vi "Data Tag Type to SysLink Type.vi"(11 "Data Tag Type":T2) -> (3 "data type":T1=enum."U64" caption="Systeme Link Data Type")   [LabVIEW 2015, in "SystemLink File configuration.lvclass"]
doc: "Converts Data Tag Type.ctl to the correct System Link data type. This is used to convert the user selected data type to a data type that system link can use."
uses:
  SystemLink File configuration.lvclass
  Data Tag Type.ctl
  <vilib>/Skyline/Tag/Shared/typedefs/DataType.ctl
  <vilib>/Skyline/Tag/Shared/NI Skyline Tag.lvlib
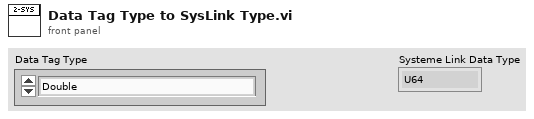
[diagram p1: front panel]
types:
  T1 = typedef "NI Skyline Tag.lvlib/DataType.ctl" = enum32{"Double", "I32", "String", "Boolean", "U64", "Timestamp"}
  T2 = typedef "SystemLink File configuration.lvclass/Data Tag Type.ctl" = enum16{"Double", "Single", "I32", "I16", "I8", "U64", "U32", "U16", "U8", "Boolean", "String", "Timestamp"}
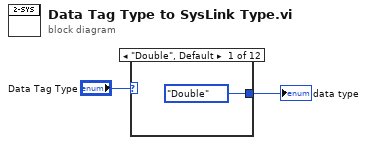
[diagram p0: block diagram]
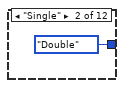
[diagram p2: hidden frame]
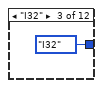
[diagram p3: hidden frame]
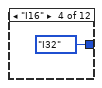
[diagram p4: hidden frame]
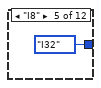
[diagram p5: hidden frame]
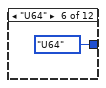
[diagram p6: hidden frame]
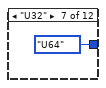
[diagram p7: hidden frame]
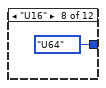
[diagram p8: hidden frame]
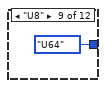
[diagram p9: hidden frame]
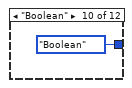
[diagram p10: hidden frame]
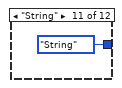
[diagram p11: hidden frame]
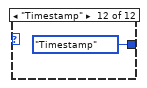
[diagram p12: hidden frame]
diagram:
  n1 = case shown="\"Double\", Default" "Data Tag Type" {
    tunnel: [DataType."Double" ("data type") DataType."Double" ("data type") DataType."I32" ("data type") DataType."I32" ("data type") DataType."I32" ("data type") DataType."U64" ("data type") DataType."U64" ("data type") DataType."U64" ("data type") DataType."U64" ("data type") DataType."Boolean" ("data type") DataType."String" ("data type") DataType."Timestamp" ("data type")] -> w1
    frame "Double", Default {
    }
    frame "Single" {
    }
    frame "I32" {
    }
    frame "I16" {
    }
    frame "I8" {
    }
    frame "U64" {
    }
    frame "U32" {
    }
    frame "U16" {
    }
    frame "U8" {
    }
    frame "Boolean" {
    }
    frame "String" {
    }
    frame "Timestamp" {
    }
  }
  "data type" <- w1
